vi "Header Column FGV.vi"(6 "Column initilization":string[](array[string])=["Time", "Throttle % ", "Speed Summary", "Torque Summary", "Power", "Gear Ratio", "Engine Speed", "Engine Torque", "L Speed", "R Speed", "H Speed", "L Torque ", "R Torque ", "H Torque ", "Intercooler_In_T", "Intercooler_Out_T", "Exhaust_T", "Oil_T", "Coolant_Inlet_T", "Coolant_Outlet_T", "Basement_T", "T Spare 1", "T Spare 2", "T Spare 3", "T Spare 4", "T Spare 5", "T Spare 6", "T Spare 7", "T Spare 8", "Coolant-In_P", "Coolant-Out_P", "Exhaust_P", "Oil_P", "Intercooler-In_P", "Intercooler-Out_P", "Misc_P ", "P Spare 1", "P Spare 2", "P Spare 3", "P Spare 4", "Engine RPM "], 7 "Command":T1(ring), 8 "error in (no error)":errorcluster, 9 "Column Header":string[](array[string])=["Time", "Throttle % ", "Speed Summary", "Torque Summary", "Power", "Gear Ratio", "Engine Speed", "Engine Torque", "L Speed", "R Speed", "H Speed", "L Torque ", "R Torque ", "H Torque ", "Intercooler_In_T", "Intercooler_Out_T", "Exhaust_T", "Oil_T", "Coolant_Inlet_T", "Coolant_Outlet_T", "Basement_T", "T Spare 1", "T Spare 2", "T Spare 3", "T Spare 4", "T Spare 5", "T Spare 6", "T Spare 7", "T Spare 8", "Coolant-In_P", "Coolant-Out_P", "Exhaust_P", "Oil_P", "Intercooler-In_P", "Intercooler-Out_P", "Misc_P ", "P Spare 1", "P Spare 2", "P Spare 3", "P Spare 4", "Engine RPM "], 11 "File Path":path) -> (0 "error out":errorcluster, 1 "Column Header":string[](array[string])=["Time", "Throttle % ", "Speed Summary", "Torque Summary", "Power", "Gear Ratio", "Engine Speed", "Engine Torque", "L Speed", "R Speed", "H Speed", "L Torque ", "R Torque ", "H Torque ", "Intercooler_In_T", "Intercooler_Out_T", "Exhaust_T", "Oil_T", "Coolant_Inlet_T", "Coolant_Outlet_T", "Basement_T", "T Spare 1", "T Spare 2", "T Spare 3", "T Spare 4", "T Spare 5", "T Spare 6", "T Spare 7", "T Spare 8", "Coolant-In_P", "Coolant-Out_P", "Exhaust_P", "Oil_P", "Intercooler-In_P", "Intercooler-Out_P", "Misc_P ", "P Spare 1", "P Spare 2", "P Spare 3", "P Spare 4", "Engine RPM "])   [LabVIEW 2018]
doc: "This Subvi usde for CSV Initialize ,Read, Write and close.\nIntilise case; we check File avaliblity in not found create csv file\nRead Case ; Read data from csv file"
uses:
  <vilib>/Utility/file.llb/Write Delimited Spreadsheet (string).vi
  <vilib>/Utility/file.llb/Read Delimited Spreadsheet (string).vi
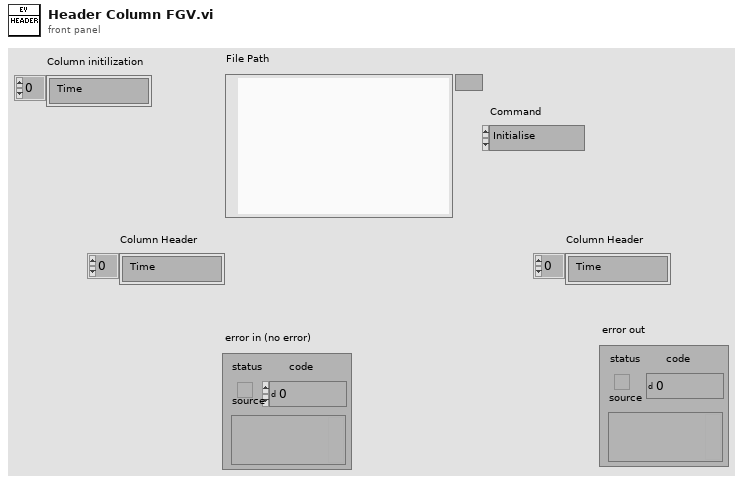
[diagram p1: front panel]
types:
  T1 = enum16{"Initialise", "Read Data", "Write Data", "Close"}
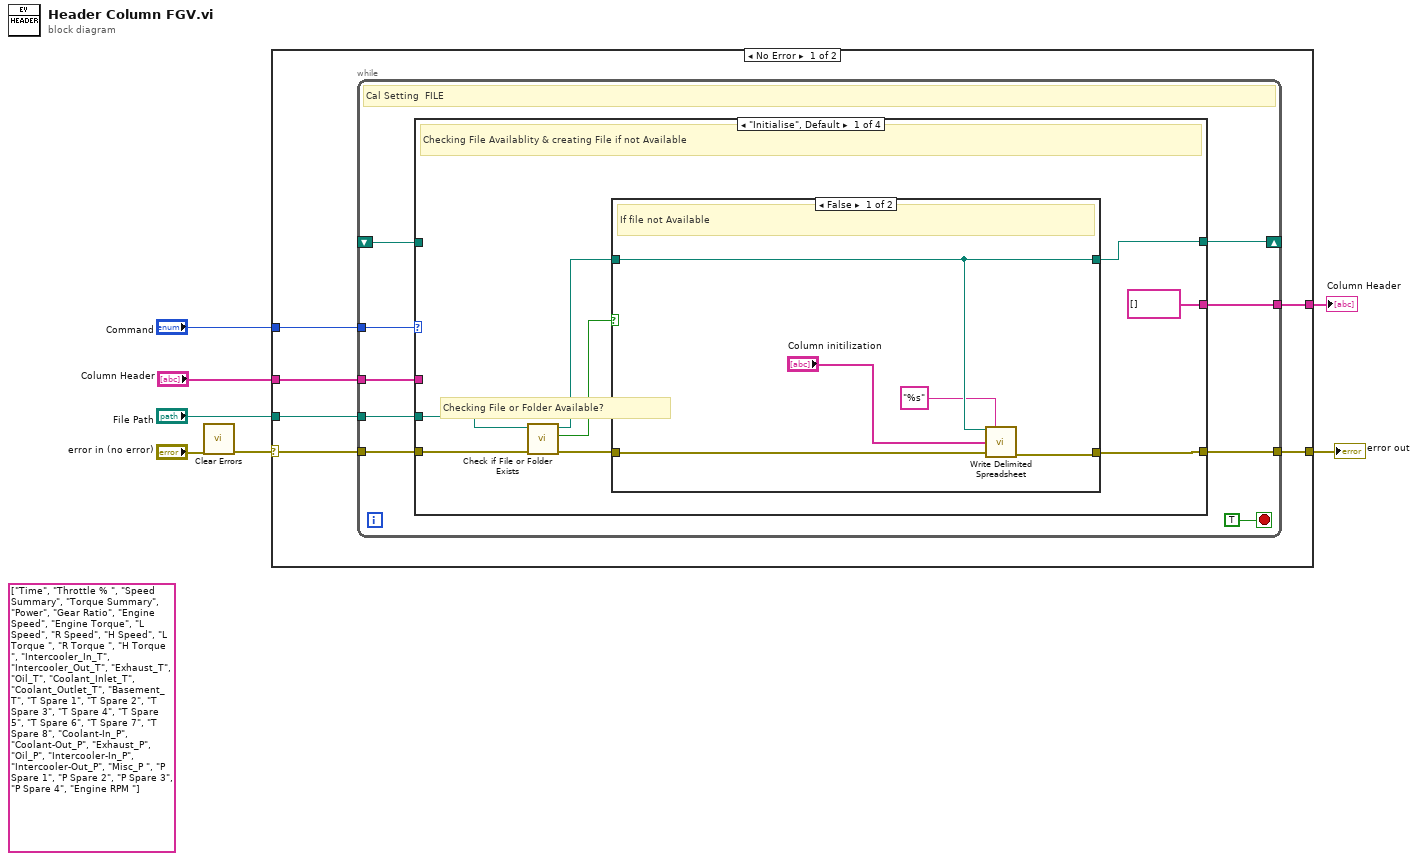
[diagram p0: block diagram]
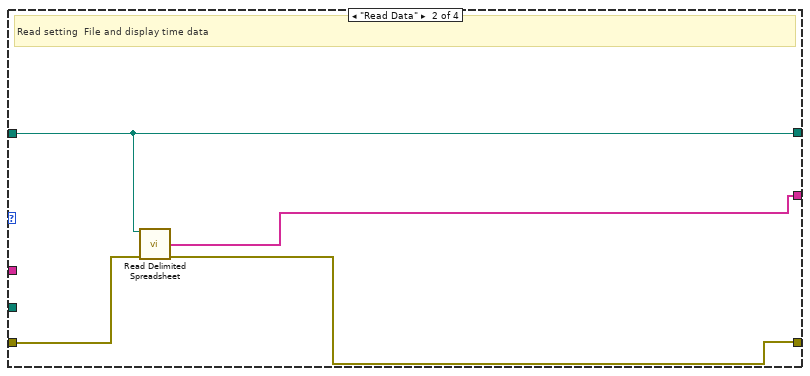
[diagram p3: hidden frame]
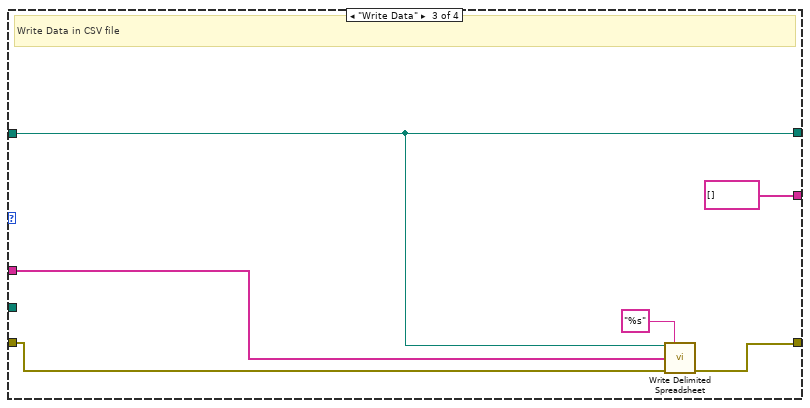
[diagram p4: hidden frame]
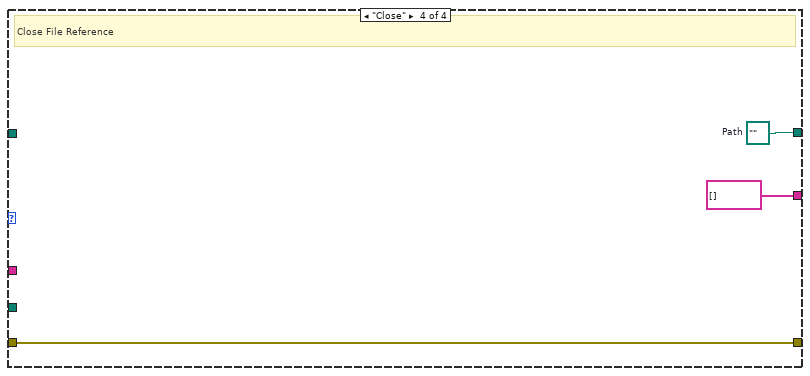
[diagram p5: hidden frame]
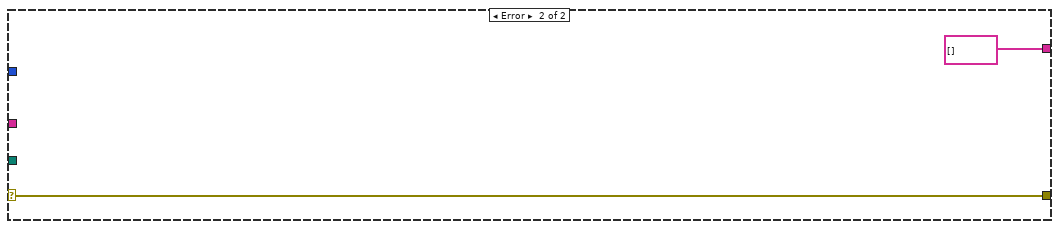
[diagram p6: hidden frame]
diagram:
  (unwired) string[] ["Time", "Throttle % ", "Speed Summary", "Torque Summary", "Power", "Gear Ratio", "Engine Speed", "Engine Torque", "L Speed", "R Speed", "H Speed", "L Torque ", "R Torque ", "H Torque ", "Intercooler_In_T", "Intercooler_Out_T", "Exhaust_T", "Oil_T", "Coolant_Inlet_T", "Coolant_Outlet_T", "Basement_T", "T Spare 1", "T Spare 2", "T Spare 3", "T Spare 4", "T Spare 5", "T Spare 6", "T Spare 7", "T Spare 8", "Coolant-In_P", "Coolant-Out_P", "Exhaust_P", "Oil_P", "Intercooler-In_P", "Intercooler-Out_P", "Misc_P ", "P Spare 1", "P Spare 2", "P Spare 3", "P Spare 4", "Engine RPM "] ("Column Header")
  n1 = call <vilib>:"Clear Errors.vi"("error in (no error)"="error in (no error)") -> ("error out"=w3:errorcluster)  [unwired: 5 in, 1 out]
  n2 = case shown="No Error" w3 {
    selector: w3 -> [w12 w52]
    tunnel: [w11 w52] -> w6
    tunnel: "Command" -> [w13 _]
    tunnel: "File Path" -> [w10 _]
    tunnel: [w9 string[] [] ("Column Header")] -> w1
    tunnel: "Column Header" -> [w8 _]
    frame No Error {
      n3 = while {
        shift-right: [w17] -> _
        shift-left: _ -> [w16]
        tunnel: w13 -> [w21]
        tunnel: w12 -> [w20]
        tunnel: [w19] -> w11
        tunnel: w10 -> [w18]
        tunnel: [w15] -> w9
        tunnel: w8 -> [w14]
        stop <- TRUE stop-if-true
        # "Cal Setting  FILE"
        n4 = case shown="\"Initialise\", Default" w21 {
          tunnel: w20 -> [w30 w40 w46 w50]
          tunnel: [w24 w39 w45 w50] -> w19
          tunnel: w18 -> [w29 _ _ _]
          tunnel: [w27 w41 w44 w49] -> w17
          tunnel: w16 -> [_ w41 w44 _]
          tunnel: [string[] [] ("Column Header") w38 string[] [] ("Column Header") string[] [] ("Column Header")] -> w15
          tunnel: w14 -> [_ _ w43 _]
          frame "Initialise", Default {
            # "Checking File or Folder Available?"
            # "Checking File Availablity & creating File if not Available"
            n5 = call <vilib>:"Check if File or Folder Exists.vi"("error in (no error)"=w30, "path"=w29) -> ("error out"=w25:errorcluster, "file or folder exists?"=w28:bool, "dup path"=w26:path)  [unwired: 7 in]
            n6 = case shown="False" w28 {
              tunnel: [w35 w37] -> w27
              tunnel: w26 -> [w35 w37]
              tunnel: w25 -> [w33 w36]
              tunnel: [w32 w36] -> w24
              frame False {
                # "If file not Available"
                n7 = call-poly <vilib>:"Write Delimited Spreadsheet.vi"("file path (dialog if empty)"=w35, "format (%s)"="%s", "1D data"="Column initilization", "error in (no error)"=w33) -> ("error out"=w32:errorcluster)  [unwired: 10 in, 1 out]
              }
              frame True {
                # "If File available"
              }
            }
          }
          frame "Read Data" {
            # "Read setting  File and display time data"
            n8 = call-poly <vilib>:"Read Delimited Spreadsheet.vi"("file path (dialog if empty)"=w41, "error in (no error)"=w40) -> ("first row"=w38:string[], "error out"=w39:errorcluster)  [unwired: 8 in, 4 out]
          }
          frame "Write Data" {
            # "Write Data in CSV file"
            n9 = call-poly <vilib>:"Write Delimited Spreadsheet.vi"("file path (dialog if empty)"=w44, "format (%s)"="%s", "1D data"=w43, "error in (no error)"=w46) -> ("error out"=w45:errorcluster)  [unwired: 10 in, 1 out]
          }
          frame "Close" {
            w49 = path ""  # Path
            # "Close File Reference"
          }
        }
      }
    }
    frame Error {
    }
  }
  "error out" <- w6
  "Column Header" <- w1
